vi "GlobeVaribles.vi"() -> ()   [LabVIEW 2016]
uses:
  Continuous Operations.ctl
panel:
  in  "1#":string
  out "记录时间":string
  out "StartSaveTRIG":bool
  out "DAQ Data":dbl[](array[numeric])
  out "save error":bool
  in  "CfgPara":T1={"ParaName"=["ChanType", "ChanName", "ChanAlias", "Unit", "Use", "SampleRate", "FilterFreq", "SlopeA", "InterceptB", "SampMax", "SampMin", "AlarmMax", "AlarmMin", "Formula"], "dfltValue"=["AI", "", "", "", "false", "1000", "100", "1", "0", "10", "-10", "Inf", "-Inf", ""]}
  in  "Status":T2
  in  "SaveInfo":string
  in  "CFilePath":string
  in  "SFilePath":string
  out "Sample?":bool
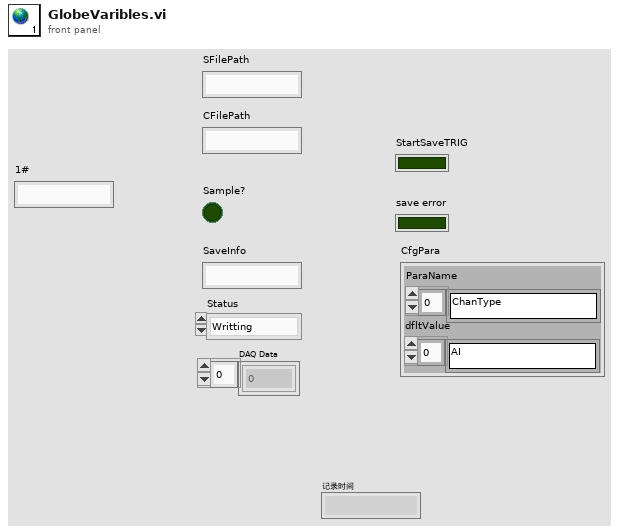
[diagram p1: front panel]
types:
  T1 = cluster{"ParaName":string[], "dfltValue":string[]}
  T2 = typedef "Continuous Operations.ctl" = enum16{"Writting", "Pause", "Stop"}
diagram:
